vi "NewClimbWeight.vi"   [LabVIEW 2013]
uses:
  State Machine Enum.ctl
  <vilib>/Rock Robotics/WPI/Solenoid/WPI_SolenoidSetEnum.vi
  <vilib>/Rock Robotics/WPI/Solenoid/WPI_SolenoidValue.ctl
types:
  T1 = typedef "State Machine Enum.ctl" = enum16{"Init", "Actuate", "Retract"}
  T2 = typedef "WPI_SolenoidValue.ctl" = enum16{"Off", "On", "Forward", "Reverse"}
  T3 = typedef "WPI_SolenoidDevRef.ctl" = cluster{"DevStatus":errorcluster, "Solenoid Module":T4, "Forward Solenoid Channel":T5, "Reverse Solenoid Channel":T5}
  T4 = typedef "FPGA_TypedefSolenoidModule.ctl" = enum16{"Solenoid Module 1", "Solenoid Module 2"}
  T5 = typedef "WPI_SolenoidChannel.ctl" = enum8{"Solenoid 1", "Solenoid 2", "Solenoid 3", "Solenoid 4", "Solenoid 5", "Solenoid 6", "Solenoid 7", "Solenoid 8", "Invalid"}
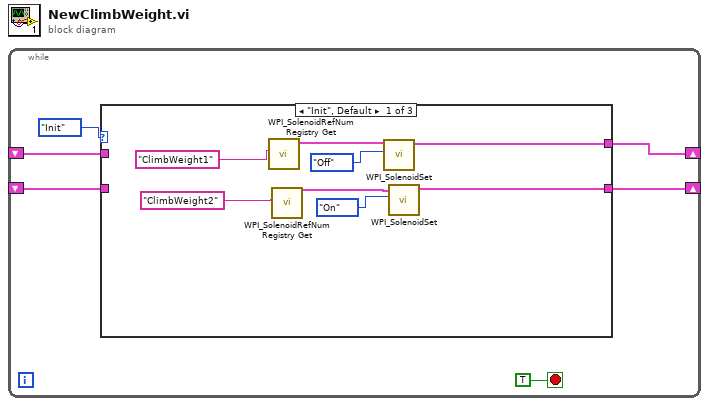
[diagram p0: block diagram]
diagram:
  n1 = while {
    shift-right: [w4] -> _
    shift-left: _ -> [w2]
    shift-right: [w3] -> _
    shift-left: _ -> [w1]
    stop <- TRUE stop-if-true
    n2 = case shown="\"Init\", Default" State_Machine_Enum."Init" ("Enum") {
      tunnel: [w8 _ _] -> w4
      tunnel: [w7 _ _] -> w3
      tunnel: w2 -> [_ _ _]
      tunnel: w1 -> [_ _ _]
      frame "Init", Default {
        n3 = call <vilib>:"WPI_SolenoidRefNum Registry Get.vi"("refnum name"="ClimbWeight1") -> ("SolenoidDevRef"=w9:T3)  [unwired: 9 in, 1 out]
        n4 = call <vilib>:"WPI_SolenoidRefNum Registry Get.vi"("refnum name"="ClimbWeight2") -> ("SolenoidDevRef"=w12:T3)  [unwired: 9 in, 1 out]
        n5 = call-poly <vilib>:"WPI_SolenoidSet.vi"("Value"=WPI_SolenoidValue."Off", "SolenoidDevRef"=w9) -> ("SolenoidDevRef"=w8:T3)  [unwired: 8 in, 1 out]
        n6 = call-poly <vilib>:"WPI_SolenoidSet.vi"("Value"=WPI_SolenoidValue."On", "SolenoidDevRef"=w12) -> ("SolenoidDevRef"=w7:T3)  [unwired: 8 in, 1 out]
      }
      frame "Actuate" {
      }
      frame "Retract" {
      }
    }
  }
